vi "Decrement.vi"(8 "error in (no error)":errorcluster, 10 "Step (1)":i32=1, 11 "LargeScrollbar in":refnum<class "LargeScrollbar.lvclass">) -> (0 "error out":errorcluster)   [LabVIEW 2015, in "LargeScrollbar.lvclass"]
doc: "<b> </b> <b> </b>\n©2016 Q Software Innovations, LLC (QSI)\nwritten by Quentin Alldredge\nproduced in LabVIEW 2015\n\nsupport@qsoftwareinnovations.com\nwww.qsoftwareinnovations.com\n\nAll rights reserved.\n\nRedistribution and use in source and binary forms, with or without modification, are permitted provided that the following conditions are met:\n\n * Redistributions of source code must retain the above copyright notice, this list of conditions and the following disclaimer.\n * Redistributions in binary form must reproduce the above copyright notice, this list of conditions and the following disclaimer in the documentation and/or other materials provided with the distribution.\n * Neither the name of Q Software Innovations, LLC. nor the names of its contributors may be used to endorse or promote products derived from this software without specific prior written permission.\n\nTHIS SOFTWARE IS PROVIDED BY THE COPYRIGHT HOLDERS AND CONTRIBUTORS \"AS IS\" AND ANY EXPRESS OR IMPLIED WARRANTIES, INCLUDING, BUT NOT LIMITED TO, THE IMPLIED WARRANTIES OF MERCHANTABILITY AND FITNESS FOR A PARTICULAR PURPOSE ARE DISCLAIMED. IN NO EVENT SHALL THE COPYRIGHT OWNER OR CONTRIBUTORS BE LIABLE FOR ANY DIRECT, INDIRECT, INCIDENTAL, SPECIAL, EXEMPLARY, OR CONSEQUENTIAL DAMAGES (INCLUDING, BUT NOT LIMITED TO, PROCUREMENT OF SUBSTITUTE GOODS OR SERVICES; LOSS OF USE, DATA, OR PROFITS; OR BUSINESS INTERRUPTION) HOWEVER CAUSED AND ON ANY THEORY OF LIABILITY, WHETHER IN CONTRACT, STRICT LIABILITY, OR TORT (INCLUDING NEGLIGENCE OR OTHERWISE) ARISING IN ANY WAY OUT OF THE USE OF THIS SOFTWARE, EVEN IF ADVISED OF THE POSSIBILITY OF SUCH DAMAGE."
uses:
  LargeScrollbar.lvclass
  Direction.ctl
  LargeScrollbar.lvclass/LargeScrollbar.ctl
  Write Direction.vi
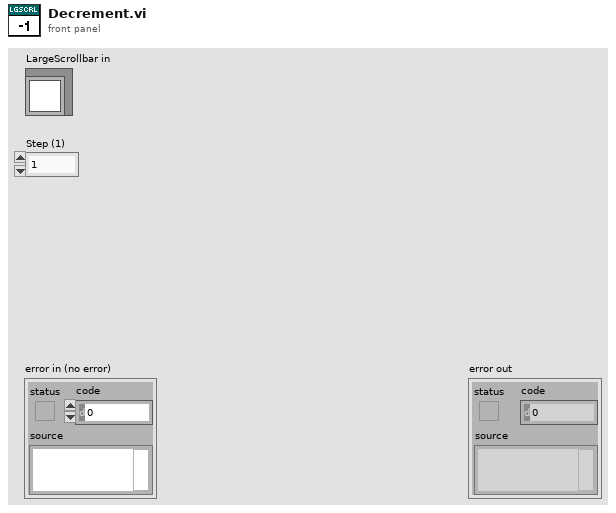
[diagram p1: front panel]
types:
  T1 = typedef "LargeScrollbar.lvclass/Direction.ctl" = enum16{"Decrement", "Increment"}
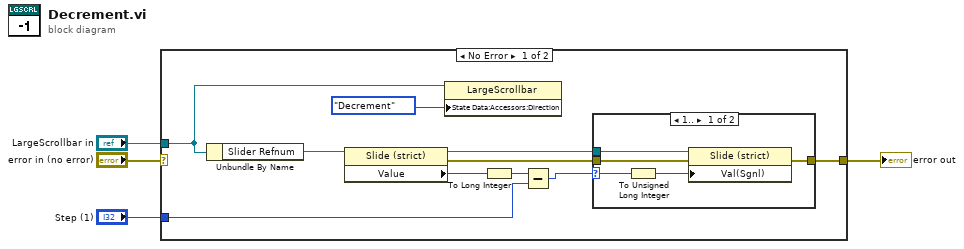
[diagram p0: block diagram]
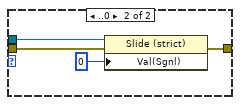
[diagram p2: hidden frame]
diagram:
  n1 = case shown="No Error" "error in (no error)" {
    selector: "error in (no error)" -> [_ w24]
    tunnel: [w11 w24] -> w3
    tunnel: "LargeScrollbar in" -> [w5 _]
    tunnel: "Step (1)" -> [w9 _]
    frame No Error {
      n2 = Unbundle By Name(w5) -> ("Slider Refnum"=w14:refnum<vi>)
      n3 = property class="Slide (strict)"(reference=w14) -> (reference out=w13:refnum<vi>, error out=w12:errorcluster, "Value"=w10:u32)  [unwired: 1 in]
      n4 = property class="LargeScrollbar"(reference=w5, "State Data:Accessors:Direction"=Direction."Decrement" ("Direction")) -> ()  [unwired: 1 in, 2 out]
      n5 = To Long Integer(number=w10) -> (32bit integer=w7:i32)
      n6 = Subtract(x=w7, y=w9) -> (x-y=w8:i32)
      n7 = case shown="1.." w8 {
        selector: w8 -> [w16 _]
        tunnel: w13 -> [w19 w23]
        tunnel: w12 -> [w18 w22]
        tunnel: [w17 w21] -> w11
        frame 1.. {
          n8 = To Unsigned Long Integer(number=w16) -> (unsigned 32bit integer=w15:u32)
          n9 = property class="Slide (strict)"(reference=w19, error in=w18, "Val(Sgnl)"=w15) -> (error out=w17:errorcluster)  [unwired: 1 out]
        }
        frame ..0 {
          n10 = property class="Slide (strict)"(reference=w23, error in=w22, "Val(Sgnl)"=u32 0 ("Value (Signaling)")) -> (error out=w21:errorcluster)  [unwired: 1 out]
        }
      }
    }
    frame Error {
    }
  }
  "error out" <- w3
